vi "Read Product.vi"(8 "error in (no error)":errorcluster, 11 "Creator in":refnum<class "Creator.lvclass">) -> (0 "error out":errorcluster, 2 "Product":refnum<class "Product.lvclass">, 3 "Creator out":refnum<class "Creator.lvclass">)   [LabVIEW 2020, in "FactoryMethod.lvlib" / "FactoryMethodLazyEvaluation.lvlib" / "Creator.lvclass"]
uses:
  Creator.lvclass
  Product/Product.lvclass
  Creator.lvclass/Creator.ctl
  TypeDef/privateDataDVR.ctl
  TypeDef/privateData.ctl
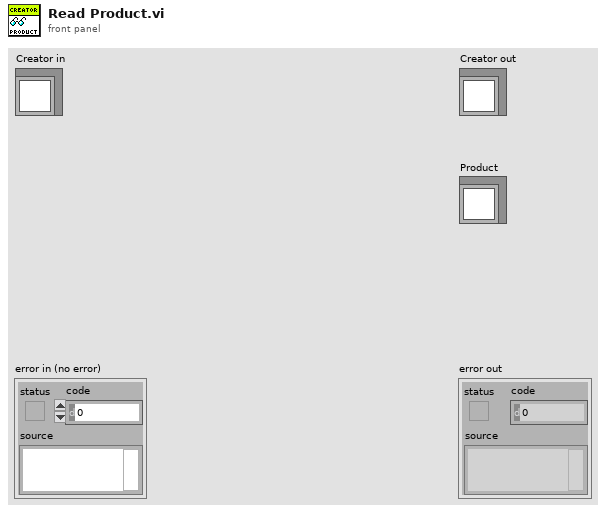
[diagram p1: front panel]
types:
  T1 = typedef "FactoryMethod.lvlib/FactoryMethodLazyEvaluation.lvlib/Creator.lvclass/privateDataDVR.ctl" = refnum<data-value>
  T2 = typedef "FactoryMethod.lvlib/FactoryMethodLazyEvaluation.lvlib/Creator.lvclass/privateData.ctl" = cluster{"Product":refnum<class "Product.lvclass">}
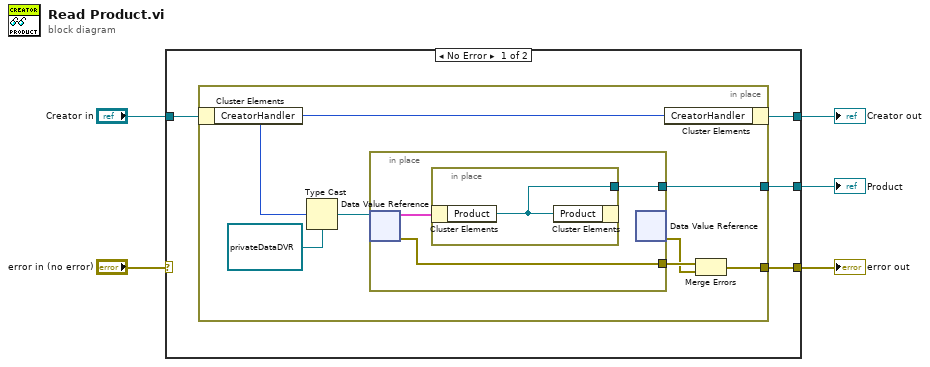
[diagram p0: block diagram]
diagram:
  n1 = case shown="No Error" "error in (no error)" {
    selector: "error in (no error)" -> [_ w22]
    tunnel: [w8 w22] -> w4
    tunnel: [w6 w21] -> w2
    tunnel: "Creator in" -> [w7 w21]
    tunnel: [w9 _] -> w1
    frame No Error {
      n2 = in-place {
        in-place-border: [w14] -> w9
        in-place-border: [w10] -> w8
        n3 = in-place-cluster #1(w7) -> ("CreatorHandler"=w13:u32)
        n4 = Type Cast(type=T1 refnum ("privateDataDVR"), x=w13) -> (*(type *) &x=w15:T1)
        n5 = in-place {
          in-place-border: [w18] -> w12
          in-place-border: [w17] -> w14
          n6 = in-place-dvr #2(w15) -> (w19:T2, w18:errorcluster)
          n7 = in-place {
            in-place-border: [w20] -> w17
            n8 = in-place-cluster #3(w19) -> ("Product"=w20:refnum<class "Product.lvclass">)
            n9 = in-place-cluster #3("Product"=w20) -> ()  [unwired: 1 out]
          }
          n10 = in-place-dvr #2() -> (w11:errorcluster)  [unwired: 1 in, 1 out]
        }
        n11 = in-place-cluster #1("CreatorHandler"=w13) -> (w6:refnum<class "Creator.lvclass">)
        n12 = Merge Errors(w12, w11) -> (w10:errorcluster)
      }
    }
    frame Error {
    }
  }
  "error out" <- w4
  "Creator out" <- w2
  "Product" <- w1
